vi "ADS get no detec.vi"(8 "error in (no error)":errorcluster, 11 "ref in":u64) -> (2 "no_of_detections":i32, 3 "ref out":u64)   [LabVIEW 2024]
uses:
  dependencies_dll_release/TCV_Lib.dll
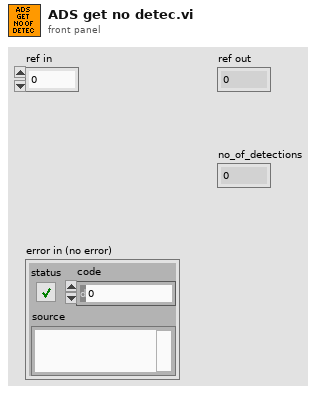
[diagram p1: front panel]
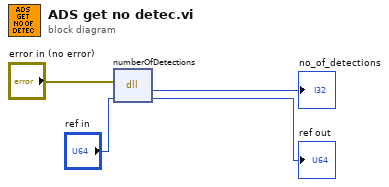
[diagram p0: block diagram]
diagram:
  n1 = dll-call lib="D:/labviewTestTCVdll/TransformCV-LabVIEW/Test/dependencies_dll_release/TCV_Lib.dll" fn="numberOfDetections"(error in="error in (no error)", "ref"="ref in") -> ("no_of_detections"=→"no_of_detections":i32, "ref"=→"ref out":u64)  [unwired: 2 in, 2 out]
